vi "Perform Action.vi"(8 "error in":errorcluster, 10 "Input":variant, 11 "HSU MCU V2 in":refnum<class "HSU MCU V2 Monitor CFG.lvclass">) -> (0 "error out":errorcluster, 2 "Output":variant, 3 "HSU MCU V2 out":refnum<class "HSU MCU V2 Monitor CFG.lvclass">)   [LabVIEW 2023, in "HSU MCU V2 Monitor CFG.lvclass"]
uses:
  HSU MCU V2 Monitor CFG.lvclass
  Attribute Selector.ctl
  MCU Selector.ctl
  3f79ec9b-441d-4d3d-ba31-e3b17ba02290.vi
  <vilib>/JDP Science/JSONtext/JSON text to Variant.vi
  <vilib>/JDP Science/JSONtext/LVClass Serializer/JSONtext LVClass Serializer.lvclass
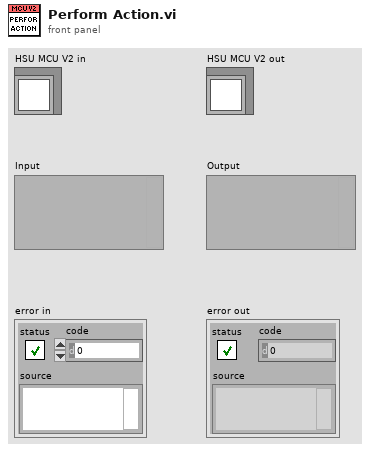
[diagram p1: front panel]
types:
  T1 = typedef "MCU Selector.ctl" = enum16{"Default", "MCU1", "MCU2", "MCU3", "MCU4", "MCU5", "MCU6", "MCU7", "MCU8"}
  T2 = typedef "Attribute Selector.ctl" = enum16{"MCU_FAULT", "MCU_STATE", "MCU_Temp_Winding", "MCU_Temp_PowerStage", "MCU_Speed", "MCU_I_REF", "MCU_ENABLE", "MCU_U_DC", "Power", "Torque"}
  T3 = cluster{"Action":enum16{"Read", "Write"}, "MCU":string, "Attribute":string, "Value":variant}
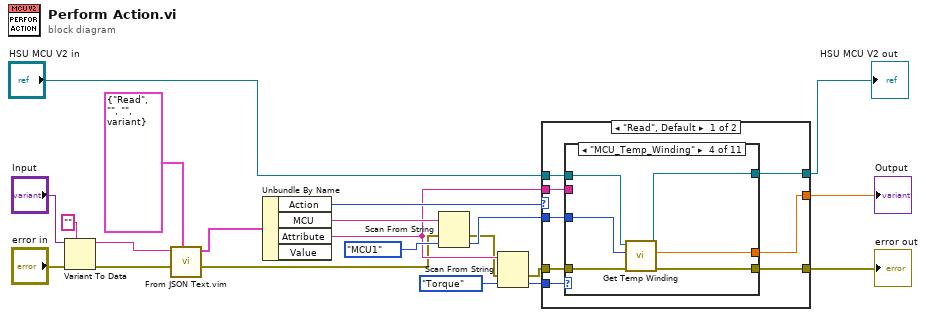
[diagram p0: block diagram]
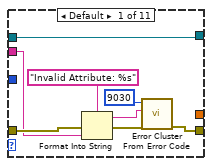
[diagram p2: hidden frame]
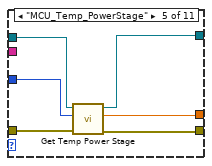
[diagram p5: hidden frame]
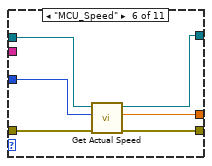
[diagram p6: hidden frame]
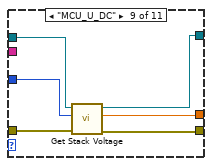
[diagram p9: hidden frame]
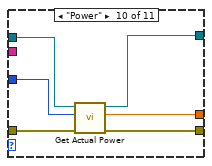
[diagram p10: hidden frame]
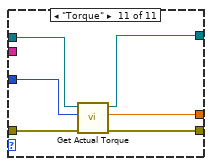
[diagram p11: hidden frame]
diagram:
  n1 = Variant To Data(error in="error in", type="", Variant="Input") -> (data=w17:string, error out=w15:errorcluster)
  n2 = call "From JSON Text.vim"("Data Type and Default Value"=T3 {"Action"=enum."Read", "MCU"="", "Attribute"="", "Value"=variant}, "error in (no error)"=w15, "JSON"=w17) -> ("error out"=w2:errorcluster, "Data out"=w13:T3)  [unwired: 7 in]
  n3 = Unbundle By Name(w13) -> ("Action"=w20:enum16{"Read", "Write"}, "MCU"=w6:string, "Attribute"=w3:string)  [unwired: 1 out]
  n4 = Scan From String(input string=w6, error in=w2, default 1=MCU_Selector."MCU1" ("MCU Selector")) -> (error out=w1:errorcluster, output 1=w4:T1)  [unwired: 2 in, 2 out]
  n5 = Scan From String(input string=w3, error in=w1, default 1=Attribute_Selector."Torque") -> (error out=w8:errorcluster, output 1=w7:T2)  [unwired: 2 in, 2 out]
  n6 = case shown="\"Read\", Default" w20 {
    tunnel: "HSU MCU V2 in" -> [w29 w82]
    tunnel: [w28 w83] -> w19
    tunnel: [w27 _] -> w12
    tunnel: [w26 w82] -> w10
    tunnel: w8 -> [w25 w83]
    tunnel: w7 -> [w24 _]
    tunnel: w4 -> [w23 _]
    tunnel: w3 -> [w22 _]
    frame "Read", Default {
      n7 = case shown="\"MCU_Temp_Winding\"" w24 {
        tunnel: w25 -> [w34 w38 w41 w47 w53 w59 w60 w62 w69 w75 w81]
        tunnel: w29 -> [w32 w39 w40 w45 w51 w55 w61 w63 w67 w72 w79]
        tunnel: [w37 w38 w41 w42 w48 w58 w60 w62 w66 w74 w80] -> w28
        tunnel: [_ _ _ w43 w49 w56 _ _ w65 w73 w77] -> w27
        tunnel: [w32 w39 w40 w44 w50 w54 w61 w63 w64 w71 w78] -> w26
        tunnel: w23 -> [_ _ _ w46 w52 w57 _ _ w68 w70 w76]
        tunnel: w22 -> [w31 _ _ _ _ _ _ _ _ _ _]
        frame Default {
          n8 = Format Into String(format string="Invalid Attribute: %s" ("error message (\"\")"), error in=w34, w31) -> (resulting string=w36:string, error out=w33:errorcluster)  [unwired: 1 in]
          n9 = call <vilib>:"Error Cluster From Error Code.vi"("error in (no error)"=w33, "error message (\"\")"=w36, "error code (0)"=9030) -> ("error out"=w37:errorcluster)  [unwired: 6 in]
        }
        frame "MCU_FAULT" {
        }
        frame "MCU_STATE" {
        }
        frame "MCU_Temp_Winding" {
          n10 = call "Get Temp Winding.vi"("error in"=w47, "MCU Selector"=w46, "HSU MCU V2 Monitor CFG in"=w45) -> ("error out"=w42:errorcluster, "Temperature"=w43:dbl, "HSU MCU V2 Monitor CFG out"=w44:refnum<class "HSU MCU V2 Monitor CFG.lvclass">)  [unwired: 6 in]
        }
        frame "MCU_Temp_PowerStage" {
          n11 = call "Get Temp Power Stage.vi"("error in"=w53, "MCU Selector"=w52, "HSU MCU V2 Monitor CFG in"=w51) -> ("error out"=w48:errorcluster, "Temperature"=w49:dbl, "HSU MCU V2 Monitor CFG out"=w50:refnum<class "HSU MCU V2 Monitor CFG.lvclass">)  [unwired: 6 in]
        }
        frame "MCU_Speed" {
          n12 = call "Get Actual Speed.vi"("error in"=w59, "MCU Selector"=w57, "HSU MCU V2 Monitor CFG in"=w55) -> ("error out"=w58:errorcluster, "Speed"=w56:dbl, "HSU MCU V2 Monitor CFG out"=w54:refnum<class "HSU MCU V2 Monitor CFG.lvclass">)  [unwired: 6 in]
        }
        frame "MCU_I_REF" {
        }
        frame "MCU_ENABLE" {
        }
        frame "MCU_U_DC" {
          n13 = call "Get Stack Voltage.vi"("error in"=w69, "MCU Selector"=w68, "HSU MCU V2 Monitor CFG in"=w67) -> ("error out"=w66:errorcluster, "Voltage DC"=w65:dbl, "HSU MCU V2 Monitor CFG out"=w64:refnum<class "HSU MCU V2 Monitor CFG.lvclass">)  [unwired: 6 in]
        }
        frame "Power" {
          n14 = call "Get Actual Power.vi"("error in"=w75, "MCU Selector"=w70, "HSU MCU V2 Monitor CFG in"=w72) -> ("error out"=w74:errorcluster, "Power"=w73:dbl, "HSU MCU V2 Monitor CFG out"=w71:refnum<class "HSU MCU V2 Monitor CFG.lvclass">)  [unwired: 5 in, 1 out]
        }
        frame "Torque" {
          n15 = call "Get Actual Torque.vi"("error in"=w81, "MCU Selector"=w76, "HSU MCU V2 Monitor CFG in"=w79) -> ("error out"=w80:errorcluster, "Torque"=w77:dbl, "HSU MCU V2 Monitor CFG out"=w78:refnum<class "HSU MCU V2 Monitor CFG.lvclass">)  [unwired: 6 in]
        }
      }
    }
    frame "Write" {
    }
  }
  "error out" <- w19
  "HSU MCU V2 out" <- w10
  "Output" <- w12
